vi "Configure Relative Offset.vi"(6 "Function":u16(ring) items=["Voltage: DC", "Voltage: AC", "Current: DC", "Current: AC", "2W Resistance", "4W Resistance", "Diode", "Capacitance", "Temperature", "Continuity", "Frequency", "Period", "Ratio", "Digitize Voltage", "Digitize Current"], 7 "Enable Offset (T: Enable)":bool=TRUE, 8 "error in (no error)":errorcluster, 9 "Manual Offset Value":dbl, 10 "Offset Value":u16(ring)=1 items=["Acquired Measurement", "Manual Offset"], 11 "VISA resource name":refnum<visa-resource-name>) -> (0 "error out":errorcluster, 3 "VISA resource name out":refnum<visa-resource-name>)   [LabVIEW 2016, in "Keithley DMM7510.lvlib"]
doc: "This VI configures the relative offset value for measurements."
uses:
  Keithley DMM7510.lvlib
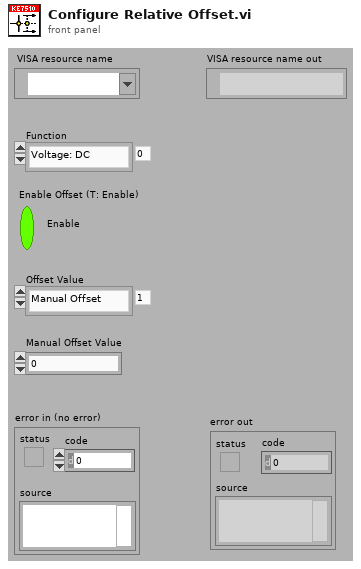
[diagram p1: front panel]
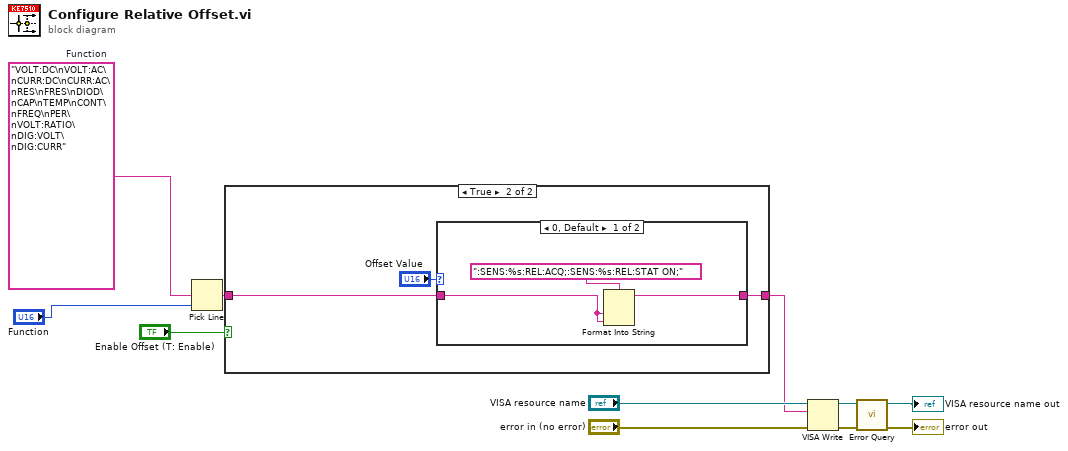
[diagram p0: block diagram]
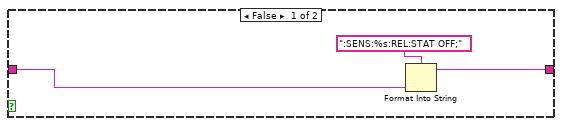
[diagram p2: hidden frame]
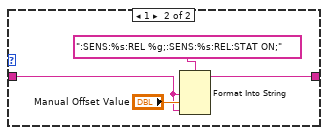
[diagram p3: hidden frame]
diagram:
  w2 = "VOLT:DC\nVOLT:AC\nCURR:DC\nCURR:AC\nRES\nFRES\nDIOD\nCAP\nTEMP\nCONT\nFREQ\nPER\nVOLT:RATIO\nDIG:VOLT\nDIG:CURR"  # Function
  n1 = Pick Line(multi-line string=w2, line index="Function") -> (output string=w3:string)  [unwired: 1 out]
  n2 = case shown="True" "Enable Offset (T: Enable)" {
    tunnel: [w14 w17] -> w5
    tunnel: w3 -> [w13 w15]
    frame False {
      n3 = Format Into String(format string=":SENS:%s:REL:STAT OFF;", w13) -> (resulting string=w14:string)  [unwired: 2 in, 1 out]
    }
    frame True {
      n4 = case shown="0, Default" "Offset Value" {
        tunnel: [w19 w24] -> w17
        tunnel: w15 -> [w18 w21]
        frame 0, Default {
          n5 = Format Into String(format string=":SENS:%s:REL:ACQ;:SENS:%s:REL:STAT ON;", w18, w18) -> (resulting string=w19:string)  [unwired: 2 in, 1 out]
        }
        frame 1 {
          n6 = Format Into String(format string=":SENS:%s:REL %g;:SENS:%s:REL:STAT ON;", w21, "Manual Offset Value", w21) -> (resulting string=w24:string)  [unwired: 2 in, 1 out]
        }
      }
    }
  }
  n7 = VISA Write(VISA resource name="VISA resource name", write buffer=w5, error in (no error)="error in (no error)") -> (VISA resource name out=w9:refnum<visa-resource-name>, error out=w6:errorcluster)  [unwired: 1 out]
  n8 = call "Error Query.vi"("error in (no error)"=w6, "VISA resource name"=w9) -> ("error out"=→"error out":errorcluster, "VISA resource name out"=→"VISA resource name out":refnum<visa-resource-name>)  [unwired: 8 out]
